vi "FTW_AppLauncher_Connection_Query.vi"(0 "FTW Actor Connector In":refnum<class "FTW-ActorConnector.lvclass">, 7 "Connection Name":string, 11 "error in (no error)":errorcluster) -> (4 "FTW Actor Connector":refnum<class "FTW-ActorConnector.lvclass">, 8 "Address":string, 14 "Roundtrip Time":dbl format="%.6fsec", 15 "error out":errorcluster)   [LabVIEW 2013]
uses:
  source/actor/Connector/FTW-ActorConnector.lvclass
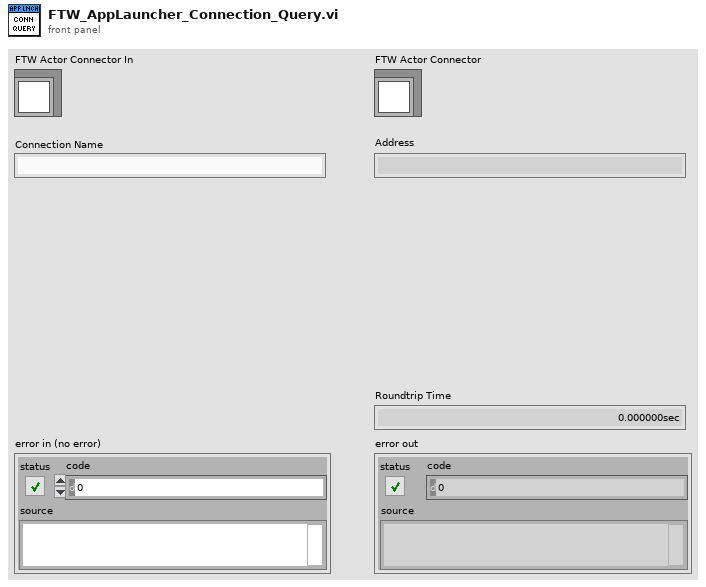
[diagram p1: front panel]
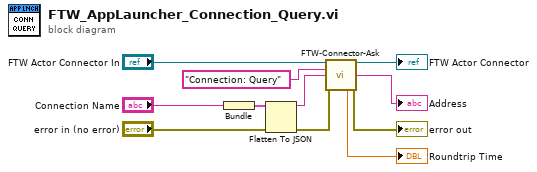
[diagram p0: block diagram]
diagram:
  n1 = Bundle("Connection Name"="Connection Name") -> (w3:cluster{"Connection Name":string})  [unwired: 1 in]
  n2 = Flatten To JSON(anything=w3, error in (no error)="error in (no error)") -> (JSON string=w2:string, 11:w4:errorcluster)  [unwired: 1 in]
  n3 = call "FTW-Connector-Ask.vi"("FTW Actor Connector"="FTW Actor Connector In", "Request Header"="Connection: Query", "Request Body"=w2, "error in"=w4) -> ("FTW Actor Connector out"=→"FTW Actor Connector":refnum<class "FTW-ActorConnector.lvclass">, "Response Body"=→"Address":string, "Roundtrip Time"=→"Roundtrip Time":dbl, "error out"=→"error out":errorcluster)  [unwired: 6 in, 2 out]
